vi "_emi_New Loops Linked Array.vi"(2 "Loop Enable (F)":bool, 7 "Loop indexes":u16[](array[numeric]), 9 "error in (no error)":errorcluster) -> (6 "Loop IDs":u16[](array[numeric]), 10 "error out":errorcluster)   [LabVIEW 2010]
doc: "Creates multiple new loops that are linked in such a way that if one stops, or is stopped, so do the others-"
uses:
  _emi_Loop control int action.ctl
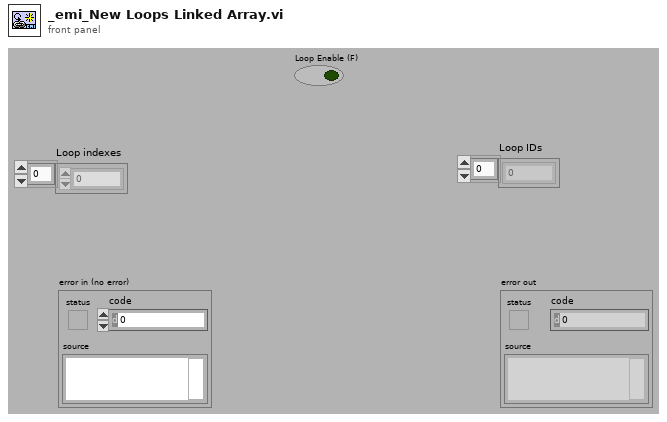
[diagram p1: front panel]
types:
  T1 = typedef "_emi_Loop control int action.ctl" = enum16{"Init index", "Get index", "Set index", "Get Size"}
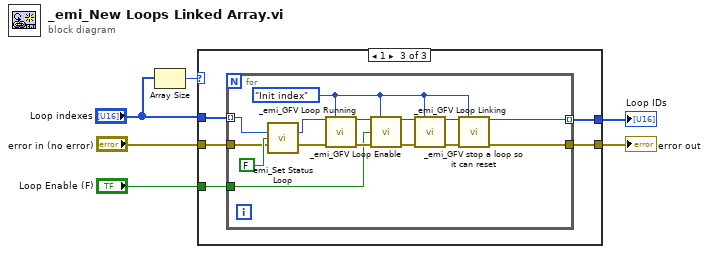
[diagram p0: block diagram]
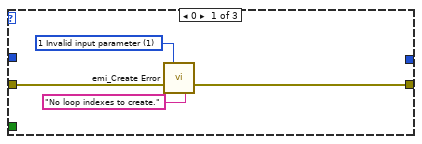
[diagram p2: hidden frame]
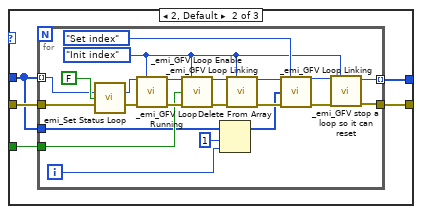
[diagram p3: hidden frame]
diagram:
  n1 = Array Size(array="Loop indexes") -> (size(s)=w3:i32)
  n2 = case shown="1" w3 {
    tunnel: "error in (no error)" -> [w9 w15 w42]
    tunnel: [w10 w14 w41] -> w5
    tunnel: "Loop Enable (F)" -> [_ w13 w40]
    tunnel: [_ w12 w39] -> w1
    tunnel: "Loop indexes" -> [_ w11 w38]
    frame 0 {
      w7 = 1 items=["0 No Error"=0, "1 Invalid input parameter"=1, "6 Generic file IO "=6, "7 File not Found"=7, "35 Generic Pring Error"=35, "37 Device not Found"=37, "39 Device Unit Error"=39, "40 Could fot Open Device"=40, "42 Generic Error"=42, "52 Unknown Message"=52, "98 Bad File type"=98, "99 Bad File Version"=99, "100 Bad Data in File"=100, "1018 Unspecefied Error"=1018, "1041 Incorrect Password"=1041, "1043 Feature not in this version"=1043, "1109 Unsuported Data type"=1109, "1444 Did not close sucessfully"=1444] ("Error Code")
      n3 = call "emi_Create Error.vi"("Error Code"=w7, "error in (no error)"=w9, "Append String(\"\")"="No loop indexes to create." ("Append String(\"\")")) -> ("error out"=w10:errorcluster)  [unwired: 12 in]
    }
    frame 2, Default {
      n4 = for {
        tunnel: w15 -> [w36]
        tunnel: [w19] -> w14
        tunnel: w13 -> [w31]
        tunnel: [w18] -> w12 mode=indexing
        tunnel: w11 -> [w30] mode=indexing
        tunnel: w11 -> [w29]
        i -> [w27]
        w16 = _emi_Loop_control_int_action."Init index" ("Action(Get Index)")
        n5 = call "emi_Set Status Loop.vi"("Loop ID in"=w30, "Running?"=FALSE, "error in (no error)"=w36) -> ("Loop ID out"=w32:u16, "error out"=w34:errorcluster)  [unwired: 11 in]
        n6 = call "_emi_GFV Loop Running.vi"("Loop Index/Numb"=w32, "Action(Get Index)"=w16, "error in (no error)"=w34) -> ("Index out"=w35:u16, "error out"=w33:errorcluster)  [unwired: 9 in, 2 out]
        n7 = call "_emi_GFV Loop Enable.vi"("Loop Index/Numb"=w35, "Action(Get Index)"=w16, "Loop enable In(T)"=w31, "error in (no error)"=w33) -> ("Index out"=w25:u16, "error out"=w26:errorcluster)  [unwired: 8 in, 2 out]
        n8 = Delete From Array(array=w29, length=1, index=w27) -> (array with subset deleted=w21:u16[])  [unwired: 1 out]
        n9 = call "_emi_GFV Loop Linking.vi"("Loop Index/Numb"=w25, "Action(Get Index)"=w16, "error in (no error)"=w26) -> ("Index out"=w22:u16, "error out"=w24:errorcluster)  [unwired: 9 in, 2 out]
        n10 = call "_emi_GFV Loop Linking.vi"("Loop Index/Numb"=w22, "Action(Get Index)"=_emi_Loop_control_int_action."Set index", "Linked indexes in"=w21, "error in (no error)"=w24) -> ("Index out"=w17:u16, "error out"=w20:errorcluster)  [unwired: 8 in, 2 out]
        n11 = call "_emi_GFV stop a loop so it can reset.vi"("Loop Index/Numb"=w17, "Action(Get Index)"=w16, "error in (no error)"=w20) -> ("Index out"=w18:u16, "error out"=w19:errorcluster)  [unwired: 9 in, 2 out]
      }
    }
    frame 1 {
      n12 = for {
        tunnel: w42 -> [w56]
        tunnel: [w46] -> w41
        tunnel: w40 -> [w51]
        tunnel: [w44] -> w39 mode=indexing
        tunnel: w38 -> [w50] mode=indexing
        w43 = _emi_Loop_control_int_action."Init index" ("Action(Get Index)")
        n13 = call "emi_Set Status Loop.vi"("Loop ID in"=w50, "Running?"=FALSE, "error in (no error)"=w56) -> ("Loop ID out"=w52:u16, "error out"=w54:errorcluster)  [unwired: 11 in]
        n14 = call "_emi_GFV Loop Running.vi"("Loop Index/Numb"=w52, "Action(Get Index)"=w43, "error in (no error)"=w54) -> ("Index out"=w55:u16, "error out"=w53:errorcluster)  [unwired: 9 in, 2 out]
        n15 = call "_emi_GFV Loop Enable.vi"("Loop Index/Numb"=w55, "Action(Get Index)"=w43, "Loop enable In(T)"=w51, "error in (no error)"=w53) -> ("Index out"=w48:u16, "error out"=w49:errorcluster)  [unwired: 8 in, 2 out]
        n16 = call "_emi_GFV Loop Linking.vi"("Loop Index/Numb"=w48, "Action(Get Index)"=w43, "error in (no error)"=w49) -> ("Index out"=w45:u16, "error out"=w47:errorcluster)  [unwired: 9 in, 2 out]
        n17 = call "_emi_GFV stop a loop so it can reset.vi"("Loop Index/Numb"=w45, "Action(Get Index)"=w43, "error in (no error)"=w47) -> ("Index out"=w44:u16, "error out"=w46:errorcluster)  [unwired: 9 in, 2 out]
      }
    }
  }
  "error out" <- w5
  "Loop IDs" <- w1
